vi "Compute.vi"(8 "error in (no error)":errorcluster, 9 "Data Channels":T1, 10 "x-var":dbl, 11 "Difference in":refnum<class "Difference.lvclass">) -> (0 "error out":errorcluster, 1 "Add'l Data Channels":T1, 3 "Difference out":refnum<class "Difference.lvclass">)   [LabVIEW 2009, in "Difference.lvclass"]
doc: "Given a data channel and an x-coordinate, compute and return one or more new data channels."
uses:
  Difference.lvclass
  Instruments/Utility Classes/Readable/Data Channels.ctl
  Instruments/Utility Classes/Readable/Data Channel.ctl
  Instruments/Utility Classes/Readable/Data Point.ctl
  Instruments/Utility Classes/Readable/Readable.lvclass
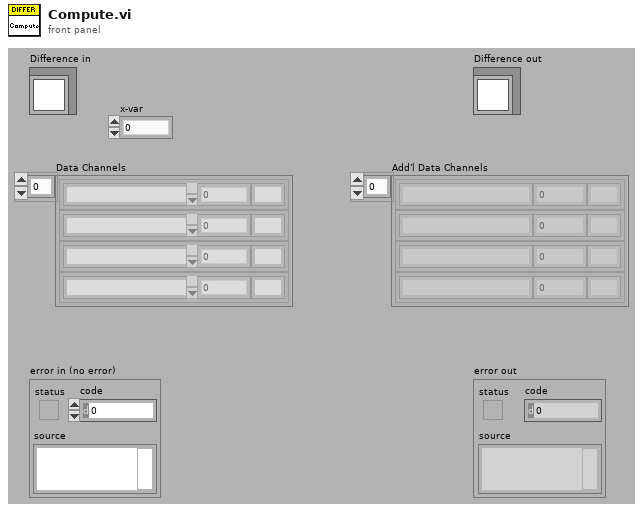
[diagram p1: front panel]
types:
  T1 = typedef "Readable.lvclass/Data Channels.ctl" = T2[]
  T2 = typedef "Readable.lvclass/Data Channel.ctl" = cluster{"Name":string, "Data Point":T3, "Unit":string}
  T3 = typedef "Readable.lvclass/Data Point.ctl" = dbl
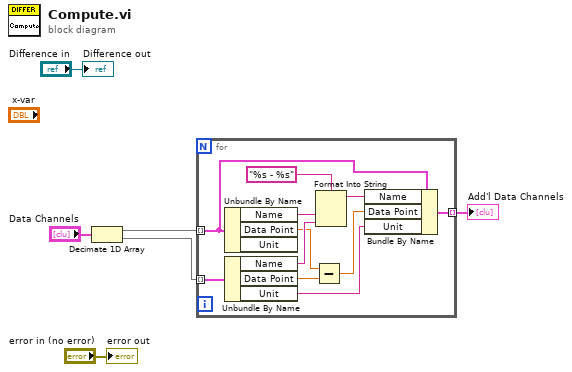
[diagram p0: block diagram]
diagram:
  n1 = Decimate 1D Array "Decimate 1D Array"("Data Channels") -> (w6:T2[], w5:T2[])
  n2 = for {
    tunnel: w6 -> [w13] mode=indexing
    tunnel: w5 -> [w17] mode=indexing
    tunnel: [w7] -> w3 mode=indexing
    n3 = Unbundle By Name(w13) -> ("Name"=w15:string, "Data Point"=w10:T3)  [unwired: 1 out]
    n4 = Unbundle By Name(w17) -> ("Name"=w14:string, "Data Point"=w9:T3, "Unit"=w12:string)
    n5 = Subtract(x=w10, y=w9) -> (x-y=w8:T3)
    n6 = Format Into String(format string="%s - %s", w15, w14) -> (resulting string=w11:string)  [unwired: 2 in, 1 out]
    n7 = Bundle By Name(cluster=w13, "Name"=w11, "Data Point"=w8, "Unit"=w12) -> (w7:T2)
  }
  "Add'l Data Channels" <- w3
  "error out" <- "error in (no error)"
  "Difference out" <- "Difference in"
